vi "Fit Transform.vi"(7 "Type X":T1(ring), 8 "error in (no error)":errorcluster caption="entrée d'erreur (pas d'erreur)", 9 "y":string[][](array[string]), 10 "X":string[][](array[string]), 11 "KNNImputer.lvclass":refnum<class "KNNImputer.lvclass">) -> (0 "error out":errorcluster caption="sortie d'erreur", 2 "Data":T2, 3 "KNNImputer.lvclass":refnum<class "KNNImputer.lvclass">)   [LabVIEW 2020, in "KNNImputer.lvclass"]
doc: "Fit to data, then transform it.\n\nFits transformer to X and y with optional parameters fit_params and returns a transformed version of X.\n\nReturns : \n\n- X_new : ndarray array of shape (n_samples, n_features_new)\nTransformed array"
uses:
  KNNImputer.lvclass
  KNNImputer.lvclass/KNNImputer.ctl
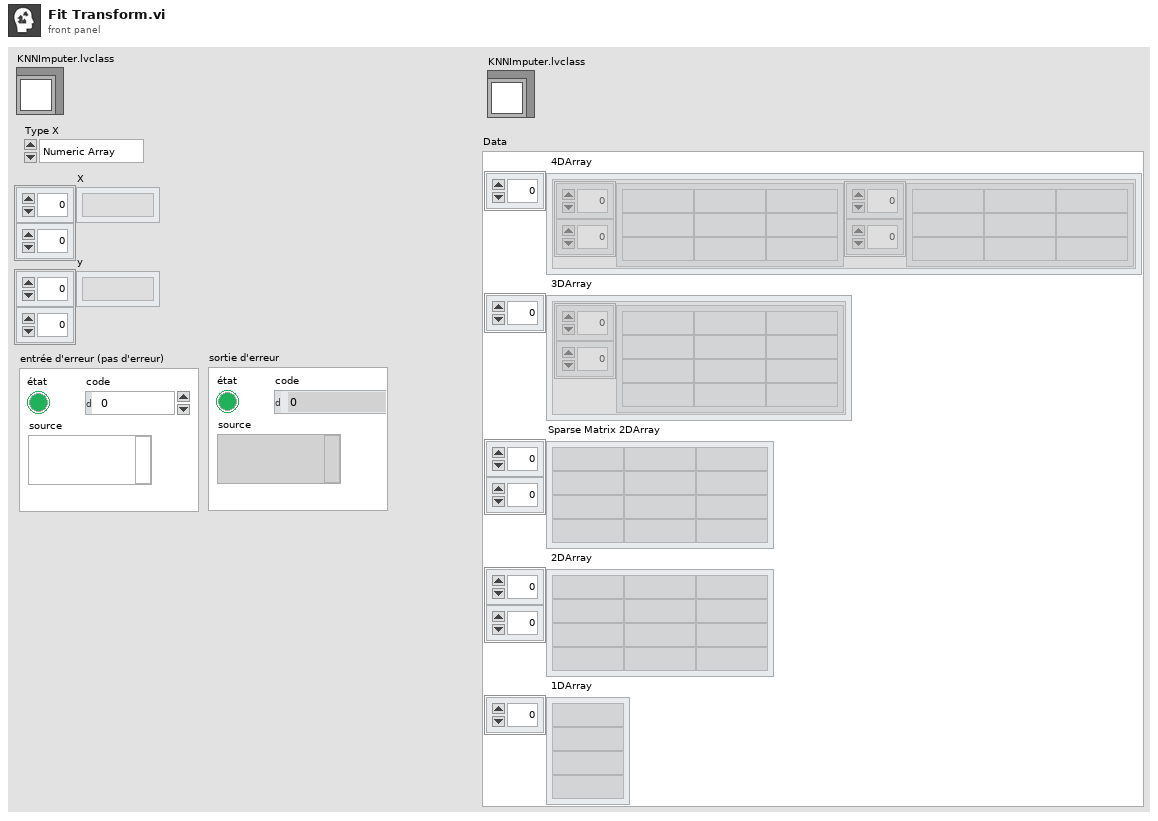
[diagram p1: front panel]
types:
  T1 = enum16{"Numeric Array", "String Array", "Sparse"}
  T2 = cluster{" 4DArray":cluster{"1":string[][], "2":string[][]}[], " 3DArray":cluster{"Tableau":string[][]}[], "Sparse Matrix 2DArray":string[][], " 2DArray":string[][], " 1DArray":string[]}
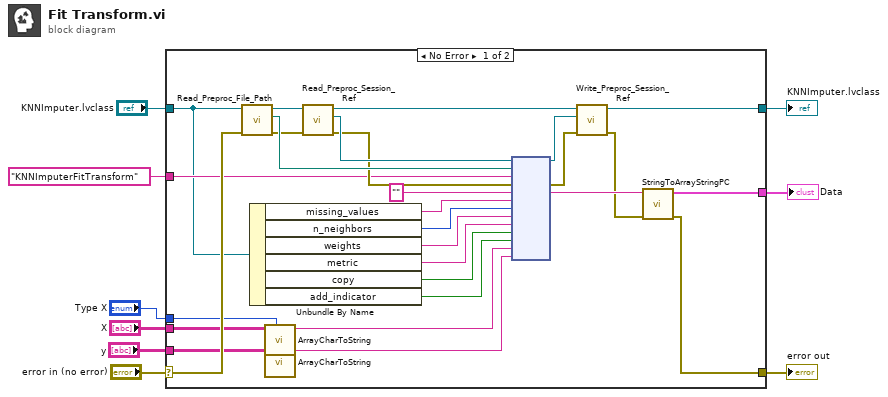
[diagram p0: block diagram]
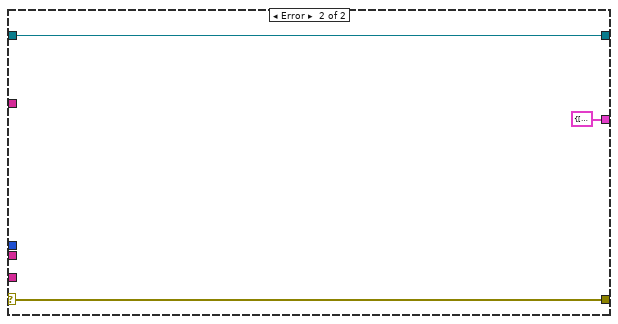
[diagram p2: hidden frame]
diagram:
  n1 = case shown="No Error" "error in (no error)" {
    selector: "error in (no error)" -> [w28 w40]
    tunnel: [w15 w40] -> w8
    tunnel: [w19 w39] -> w6
    tunnel: "KNNImputer.lvclass" -> [w26 w39]
    tunnel: "KNNImputerFitTransform" ("Fonction") -> [w27 _]
    tunnel: [w16 T2 {" 4DArray"=[], " 3DArray"=[], "Sparse Matrix 2DArray"=[], " 2DArray"=[], " 1DArray"=[]} ("Data")] -> w2
    tunnel: "X" -> [w14 _]
    tunnel: "y" -> [w12 _]
    tunnel: "Type X" -> [w10 _]
    frame No Error {
      n2 = call-dynamic "Read_Preproc_File_Path.vi"("error in (no error)"=w28, "Python in"=w26) -> ("error out"=w32:errorcluster, "File_Path"=w35:path, "Python out"=w37:refnum<class "KNNImputer.lvclass">)  [unwired: 7 in]
      n3 = Unbundle By Name(w26) -> ("missing_values"=w25:string, "n_neighbors"=w24:i32, "weights"=w23:string, "metric"=w22:string, "copy"=w21:bool, "add_indicator"=w20:bool)
      n4 = call "ArrayCharToString.vi"("Type"=w10, "TAB"=w14) -> ("Instruction"=w13:string)  [unwired: 9 in]
      n5 = call "ArrayCharToString.vi"("TAB"=w12) -> ("Instruction"=w11:string)  [unwired: 10 in]
      n6 = call-dynamic "Read_Preproc_Session_Ref.vi"("error in (no error)"=w32, "Python in"=w37) -> ("error out"=w33:errorcluster, "Session_ref"=w34:refnum<k35>, "Python out"=w36:refnum<class "KNNImputer.lvclass">)  [unwired: 7 in]
      n7 = node(w34, w35, w27, w33, "", w25, w24, w23, w22, w21, w20, w13, w11) -> (w29:refnum<k35>, w31:errorcluster, w18:string)  [unwired: 8 in, 2 out]
      n8 = call-dynamic "Write_Preproc_Session_Ref.vi"("error in (no error)"=w31, "Session_ref"=w29, "Python in"=w36) -> ("error out"=w17:errorcluster, "Python out"=w19:refnum<class "KNNImputer.lvclass">)  [unwired: 7 in]
      n9 = call "StringToArrayStringPC.vi"("sortie d'erreur"=w17, "Return value"=w18) -> ("sortie d'erreur"=w15:errorcluster, "Data"=w16:T2)  [unwired: 8 in]
    }
    frame Error {
    }
  }
  "error out" <- w8
  "KNNImputer.lvclass" <- w6
  "Data" <- w2
